vi "MarbleDispenserMk8.vi"() -> ()   [LabVIEW 2016]
uses:
  <vilib>/NXT/Block Support/NXT_InputPort.ctl
  <vilib>/NXT/Block Support/NXT_OutputPort.ctl
  <vilib>/NXT/Dual Mode Library/Sensors/Touch_Released.vi
  <vilib>/NXT/NXTIO Xnodes/NXTIONodeSubVIs/NXTStopMotors.vi
  <vilib>/NXT/NXTIO Xnodes/NXTIONodeSubVIs/NXTMotorRunDistance.vi
  <vilib>/NXT/Dual Mode Library/Waits/Wait_Num.vi
  <vilib>/NXT/Dual Mode Library/Sensors/Touch_Pressed.vi
  <vilib>/NXT/Dual Mode Library/Sensors/EV3_Color_Color.vi
  <vilib>/NXT/Dual Mode Library/Sensors/EV3_Color_Reflect.vi
  <vilib>/NXT/Subs/LVHSConnector.ctl
  <vilib>/NXT/NXTIO Xnodes/AddressXNode/NXTIOAddress.xnode
  <vilib>/NXT/NXTIO Xnodes/NXTIOXNode/NXTIO.xnode
  <vilib>/NXT/LegoClasses/BrickReference/BrickReference.lvclass
panel:
  out "Speed":dbl
  out "Color":string
  out "Distance":dbl
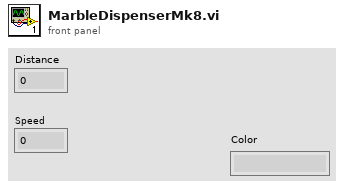
[diagram p1: front panel]
types:
  T1 = typedef "NXT_InputPort.ctl" = u32
  T2 = typedef "NXT_OutputPort.ctl" = u8
  T3 = typedef "LVHSConnector.ctl" = refnum<class "BrickReference.lvclass">
  T4 = typedef "ColorSensorColors.ctl" = enum16{"No Color", "Black", "Blue", "Green", "Yellow", "Red", "White", "Brown"}
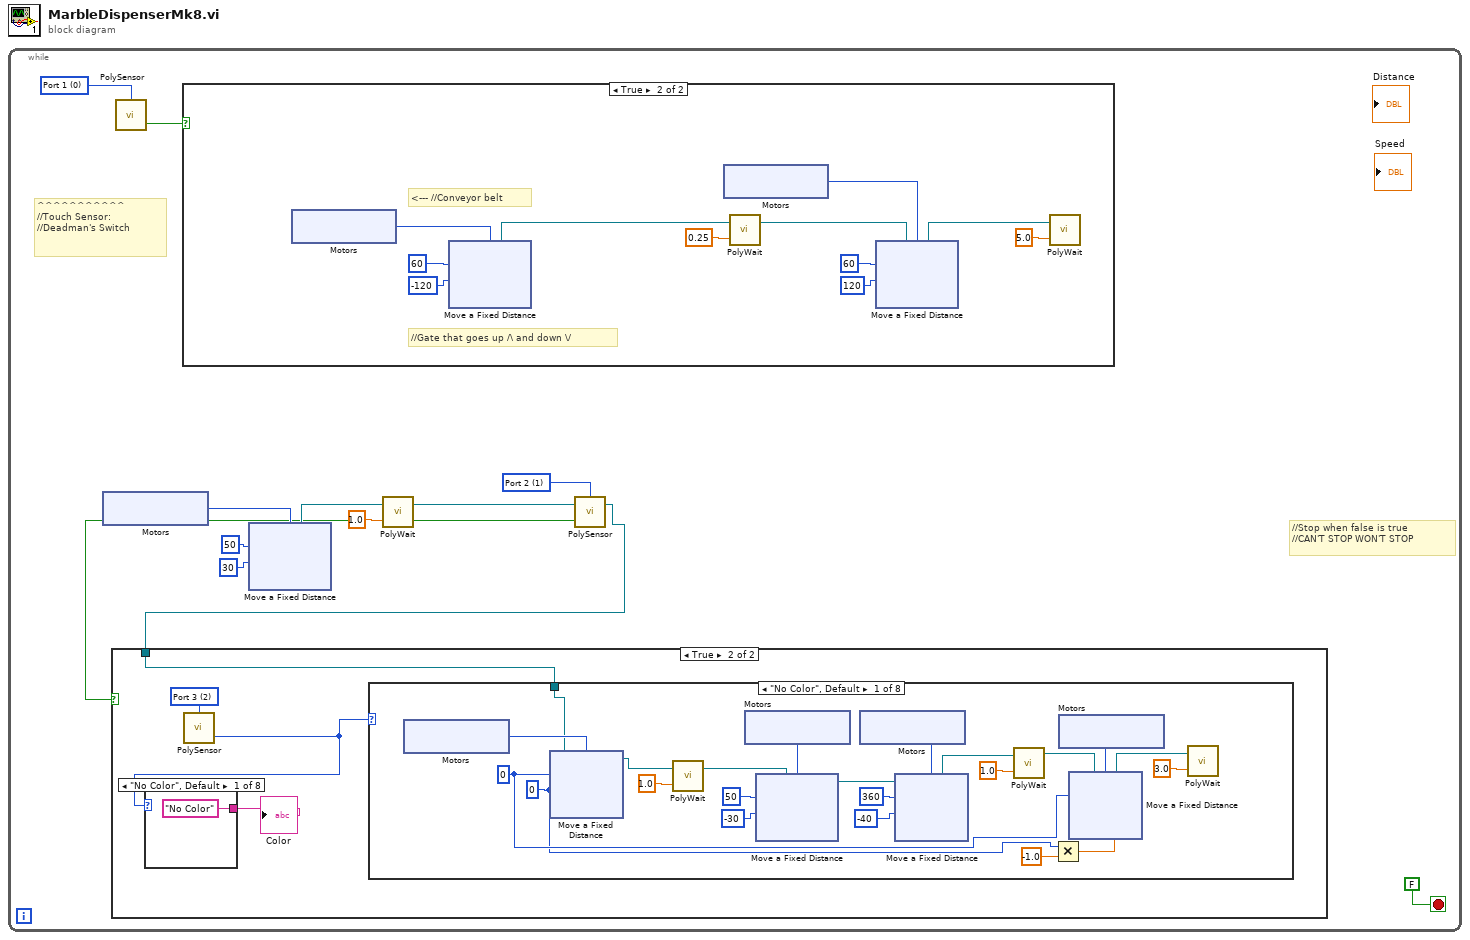
[diagram p0: block diagram]
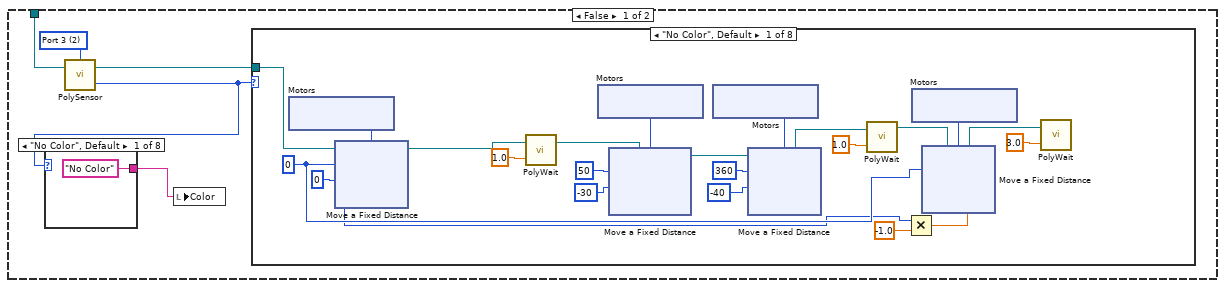
[diagram p2: hidden frame]
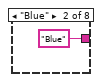
[diagram p3: hidden frame]
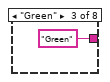
[diagram p4: hidden frame]
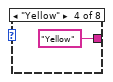
[diagram p5: hidden frame]
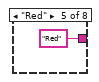
[diagram p6: hidden frame]
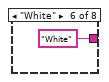
[diagram p7: hidden frame]
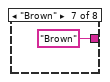
[diagram p8: hidden frame]
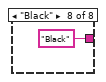
[diagram p9: hidden frame]
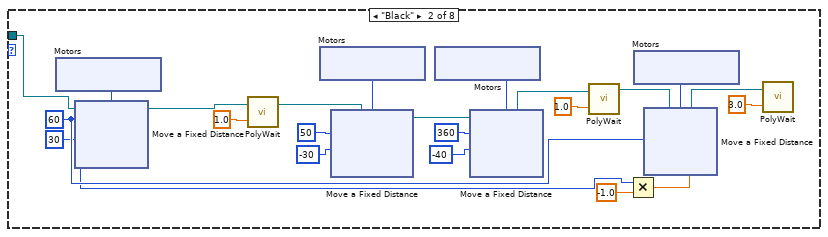
[diagram p10: hidden frame]
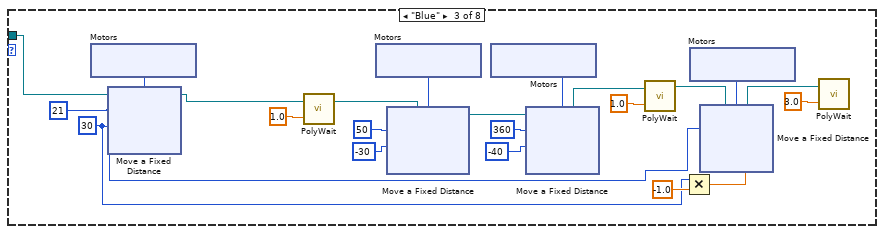
[diagram p11: hidden frame]
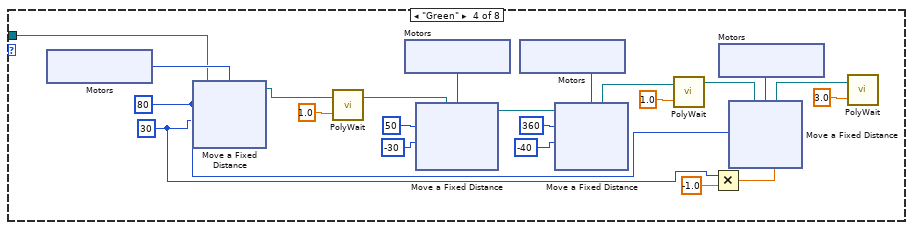
[diagram p12: hidden frame]
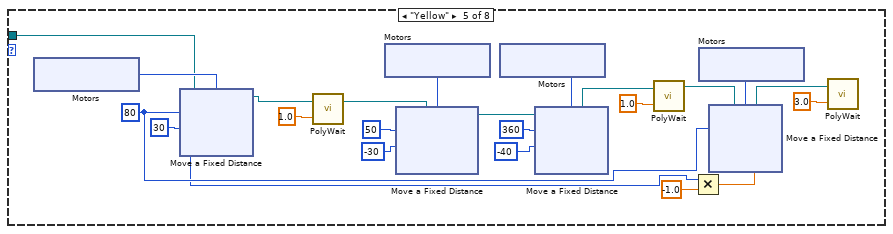
[diagram p13: hidden frame]
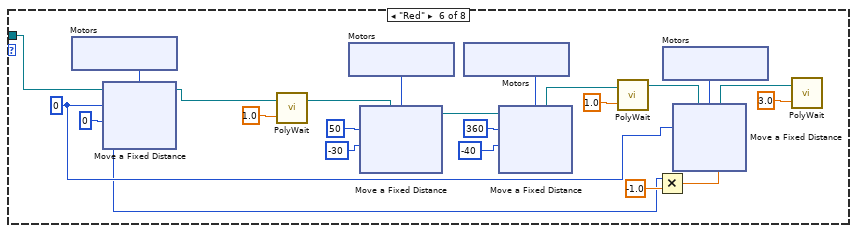
[diagram p14: hidden frame]
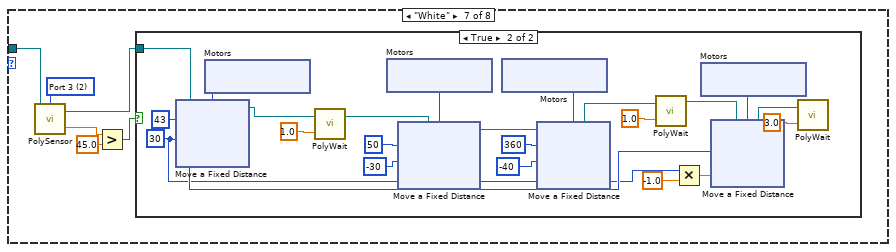
[diagram p15: hidden frame]
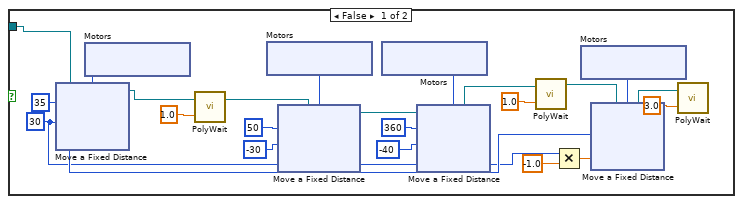
[diagram p16: hidden frame]
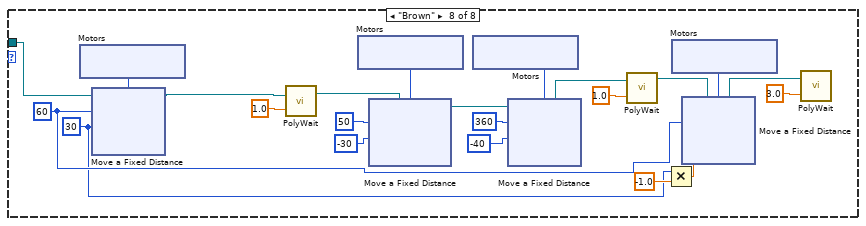
[diagram p17: hidden frame]
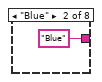
[diagram p18: hidden frame]
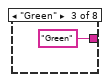
[diagram p19: hidden frame]
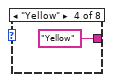
[diagram p20: hidden frame]
diagram:
  n1 = while {
    stop <- FALSE stop-if-true
    w3 = T1 1 items=["Port 1", "Port 2", "Port 3", "Port 4"] ("Port (Port 1)")
    w12 = T1 0 items=["Port 1", "Port 2", "Port 3", "Port 4"] ("Port (Port 1)")
    # "//Stop when false is true\n//CAN'T STOP WON'T STOP"
    # "^^^^^^^^^^^\n//Touch Sensor:\n//Deadman's Switch"
    n2 = xnode "Motors"() -> ("Motor"=w5:T2)
    n3 = call-poly <vilib>:"PolySensor.vi"("Port (Port 1)"=w12) -> ("Yes / No"=w10:bool)  [unwired: 2 in, 1 out]
    n4 = case shown="True" w10 {
      frame False {
        # "//This stops all the things"
        n5 = xnode "Motors"() -> ("Motor"=w1178:T2)
        n6 = xnode "Motors"() -> ("Motor"=w1177:T2)
        n7 = xnode "Stop Motors"("Motors"=w1178) -> ()  [unwired: 1 in, 1 out]
        n8 = xnode "Stop Motors"("Motors"=w1177) -> ()  [unwired: 1 in, 1 out]
      }
      frame True {
        # "//Gate that goes up /\\ and down \\/"
        # "<--- //Conveyor belt"
        n9 = xnode "Motors"() -> ("Motor"=w1197:T2)
        n10 = xnode "Move a Fixed Distance"("Speed 1"=-120, "Distance 1"=60, "Motors"=w1197) -> ("NXT/EV3"=w1200:T3)  [unwired: 1 in]
        n11 = xnode "Motors"() -> ("Motor"=w1191:T2)
        n12 = call-poly <vilib>:"PolyWait.vi"("Time (1 sec)"=0.25, "NXT/EV3"=w1200) -> ("NXT/EV3"=w1192:T3)  [unwired: 2 in]
        n13 = xnode "Move a Fixed Distance"("Speed 1"=120, "Distance 1"=60, "Motors"=w1191, "NXT/EV3"=w1192) -> ("NXT/EV3"=w1195:T3)
        n14 = call-poly <vilib>:"PolyWait.vi"("Time (1 sec)"=5.0, "NXT/EV3"=w1195) -> ()  [unwired: 2 in, 1 out]
      }
    }
    n15 = xnode "Move a Fixed Distance"("Speed 1"=30, "Distance 1"=50, "Motors"=w5) -> ("NXT/EV3"=w8:T3)  [unwired: 1 in]
    n16 = call-poly <vilib>:"PolyWait.vi"("Time (1 sec)"=1.0, "NXT/EV3"=w8) -> ("NXT/EV3"=w4:T3)  [unwired: 2 in]
    n17 = call-poly <vilib>:"PolySensor.vi"("NXT/EV3"=w4, "Port (Port 1)"=w3) -> ("Yes / No"=w2:bool, "NXT/EV3"=w1:T3)  [unwired: 1 in]
    n18 = case shown="True" w2 {
      tunnel: w1 -> [w14 w626]
      frame False {
        w17 = T1 2 items=["Port 1", "Port 2", "Port 3", "Port 4"] ("Port (Port 1)")
        n19 = call-poly <vilib>:"PolySensor.vi"("NXT/EV3"=w14, "Port (Port 1)"=w17) -> ("Detected Color"=w16:T4, "NXT/EV3"=w13:T3)  [unwired: 1 in]
        n20 = case shown="\"No Color\", Default" w16 {
          tunnel: ["No Color" "Blue" "Green" "Yellow" "Red" "White" "Brown" "Black"] -> w15
          frame "No Color", Default {
          }
          frame "Blue" {
          }
          frame "Green" {
          }
          frame "Yellow" {
          }
          frame "Red" {
          }
          frame "White" {
          }
          frame "Brown" {
          }
          frame "Black" {
          }
        }
        n21 = local write "Color"(w15) -> ()
        n22 = case shown="\"No Color\", Default" w16 {
          tunnel: w13 -> [w28 w95 w160 w227 w290 w376 w427 w560]
          frame "No Color", Default {
            w26 = i8 0 ("Speed 1")
            w27 = 0 ("Distance 1")
            n23 = xnode "Motors"() -> ("Motor"=w47:T2)
            n24 = xnode "Move a Fixed Distance"("Speed 1"=w26, "Distance 1"=w27, "Motors"=w47, "NXT/EV3"=w28) -> ("NXT/EV3"=w29:T3)
            n25 = call-poly <vilib>:"PolyWait.vi"("Time (1 sec)"=sgl 1.0, "NXT/EV3"=w29) -> ("NXT/EV3"=w42:T3)  [unwired: 2 in]
            n26 = xnode "Motors"() -> ("Motor"=w43:T2)
            n27 = xnode "Move a Fixed Distance"("Speed 1"=-30, "Distance 1"=50, "Motors"=w43, "NXT/EV3"=w42) -> ("NXT/EV3"=w32:T3)
            n28 = xnode "Motors"() -> ("Motor"=w39:T2)
            n29 = xnode "Move a Fixed Distance"("Speed 1"=i8 -40, "Distance 1"=360, "Motors"=w39, "NXT/EV3"=w32) -> ("NXT/EV3"=w40:T3)
            n30 = call-poly <vilib>:"PolyWait.vi"("Time (1 sec)"=1.0, "NXT/EV3"=w40) -> ("NXT/EV3"=w35:T3)  [unwired: 2 in]
            n31 = Multiply(x=w26, y=-1.0) -> (x*y=w30:dbl)
            n32 = xnode "Motors"() -> ("Motor"=w34:T2)
            n33 = xnode "Move a Fixed Distance"("Speed 1"=w30, "Distance 1"=w27, "Motors"=w34, "NXT/EV3"=w35) -> ("NXT/EV3"=w33:T3)
            n34 = call-poly <vilib>:"PolyWait.vi"("Time (1 sec)"=3.0, "NXT/EV3"=w33) -> ()  [unwired: 2 in, 1 out]
          }
          frame "Black" {
            w92 = i8 30 ("Speed 1")
            w93 = 60 ("Distance 1")
            n35 = xnode "Motors"() -> ("Motor"=w113:T2)
            n36 = xnode "Move a Fixed Distance"("Speed 1"=w92, "Distance 1"=w93, "Motors"=w113, "NXT/EV3"=w95) -> ("NXT/EV3"=w94:T3)
            n37 = call-poly <vilib>:"PolyWait.vi"("Time (1 sec)"=sgl 1.0, "NXT/EV3"=w94) -> ("NXT/EV3"=w108:T3)  [unwired: 2 in]
            n38 = xnode "Motors"() -> ("Motor"=w109:T2)
            n39 = xnode "Move a Fixed Distance"("Speed 1"=-30, "Distance 1"=50, "Motors"=w109, "NXT/EV3"=w108) -> ("NXT/EV3"=w98:T3)
            n40 = xnode "Motors"() -> ("Motor"=w105:T2)
            n41 = xnode "Move a Fixed Distance"("Speed 1"=i8 -40, "Distance 1"=360, "Motors"=w105, "NXT/EV3"=w98) -> ("NXT/EV3"=w106:T3)
            n42 = call-poly <vilib>:"PolyWait.vi"("Time (1 sec)"=1.0, "NXT/EV3"=w106) -> ("NXT/EV3"=w101:T3)  [unwired: 2 in]
            n43 = Multiply(x=w92, y=-1.0) -> (x*y=w96:dbl)
            n44 = xnode "Motors"() -> ("Motor"=w100:T2)
            n45 = xnode "Move a Fixed Distance"("Speed 1"=w96, "Distance 1"=w93, "Motors"=w100, "NXT/EV3"=w101) -> ("NXT/EV3"=w99:T3)
            n46 = call-poly <vilib>:"PolyWait.vi"("Time (1 sec)"=3.0, "NXT/EV3"=w99) -> ()  [unwired: 2 in, 1 out]
          }
          frame "Blue" {
            w158 = i8 30 ("Speed 1")
            w159 = 21 ("Distance 1")
            n47 = xnode "Motors"() -> ("Motor"=w179:T2)
            n48 = xnode "Move a Fixed Distance"("Speed 1"=w158, "Distance 1"=w159, "Motors"=w179, "NXT/EV3"=w160) -> ("NXT/EV3"=w161:T3)
            n49 = call-poly <vilib>:"PolyWait.vi"("Time (1 sec)"=sgl 1.0, "NXT/EV3"=w161) -> ("NXT/EV3"=w174:T3)  [unwired: 2 in]
            n50 = xnode "Motors"() -> ("Motor"=w175:T2)
            n51 = xnode "Move a Fixed Distance"("Speed 1"=-30, "Distance 1"=50, "Motors"=w175, "NXT/EV3"=w174) -> ("NXT/EV3"=w164:T3)
            n52 = xnode "Motors"() -> ("Motor"=w171:T2)
            n53 = xnode "Move a Fixed Distance"("Speed 1"=i8 -40, "Distance 1"=360, "Motors"=w171, "NXT/EV3"=w164) -> ("NXT/EV3"=w172:T3)
            n54 = call-poly <vilib>:"PolyWait.vi"("Time (1 sec)"=1.0, "NXT/EV3"=w172) -> ("NXT/EV3"=w167:T3)  [unwired: 2 in]
            n55 = Multiply(x=w158, y=-1.0) -> (x*y=w162:dbl)
            n56 = xnode "Motors"() -> ("Motor"=w166:T2)
            n57 = xnode "Move a Fixed Distance"("Speed 1"=w162, "Distance 1"=w159, "Motors"=w166, "NXT/EV3"=w167) -> ("NXT/EV3"=w165:T3)
            n58 = call-poly <vilib>:"PolyWait.vi"("Time (1 sec)"=3.0, "NXT/EV3"=w165) -> ()  [unwired: 2 in, 1 out]
          }
          frame "Green" {
            w224 = i8 30 ("Speed 1")
            w225 = 80 ("Distance 1")
            n59 = xnode "Motors"() -> ("Motor"=w245:T2)
            n60 = xnode "Move a Fixed Distance"("Speed 1"=w224, "Distance 1"=w225, "Motors"=w245, "NXT/EV3"=w227) -> ("NXT/EV3"=w226:T3)
            n61 = call-poly <vilib>:"PolyWait.vi"("Time (1 sec)"=sgl 1.0, "NXT/EV3"=w226) -> ("NXT/EV3"=w240:T3)  [unwired: 2 in]
            n62 = xnode "Motors"() -> ("Motor"=w241:T2)
            n63 = xnode "Move a Fixed Distance"("Speed 1"=-30, "Distance 1"=50, "Motors"=w241, "NXT/EV3"=w240) -> ("NXT/EV3"=w230:T3)
            n64 = xnode "Motors"() -> ("Motor"=w237:T2)
            n65 = xnode "Move a Fixed Distance"("Speed 1"=i8 -40, "Distance 1"=360, "Motors"=w237, "NXT/EV3"=w230) -> ("NXT/EV3"=w238:T3)
            n66 = call-poly <vilib>:"PolyWait.vi"("Time (1 sec)"=1.0, "NXT/EV3"=w238) -> ("NXT/EV3"=w233:T3)  [unwired: 2 in]
            n67 = Multiply(x=w224, y=-1.0) -> (x*y=w228:dbl)
            n68 = xnode "Motors"() -> ("Motor"=w232:T2)
            n69 = xnode "Move a Fixed Distance"("Speed 1"=w228, "Distance 1"=w225, "Motors"=w232, "NXT/EV3"=w233) -> ("NXT/EV3"=w231:T3)
            n70 = call-poly <vilib>:"PolyWait.vi"("Time (1 sec)"=3.0, "NXT/EV3"=w231) -> ()  [unwired: 2 in, 1 out]
          }
          frame "Yellow" {
            w291 = i8 30 ("Speed 1")
            w292 = 80 ("Distance 1")
            n71 = xnode "Motors"() -> ("Motor"=w311:T2)
            n72 = xnode "Move a Fixed Distance"("Speed 1"=w291, "Distance 1"=w292, "Motors"=w311, "NXT/EV3"=w290) -> ("NXT/EV3"=w293:T3)
            n73 = call-poly <vilib>:"PolyWait.vi"("Time (1 sec)"=sgl 1.0, "NXT/EV3"=w293) -> ("NXT/EV3"=w306:T3)  [unwired: 2 in]
            n74 = xnode "Motors"() -> ("Motor"=w307:T2)
            n75 = xnode "Move a Fixed Distance"("Speed 1"=-30, "Distance 1"=50, "Motors"=w307, "NXT/EV3"=w306) -> ("NXT/EV3"=w296:T3)
            n76 = xnode "Motors"() -> ("Motor"=w303:T2)
            n77 = xnode "Move a Fixed Distance"("Speed 1"=i8 -40, "Distance 1"=360, "Motors"=w303, "NXT/EV3"=w296) -> ("NXT/EV3"=w304:T3)
            n78 = call-poly <vilib>:"PolyWait.vi"("Time (1 sec)"=1.0, "NXT/EV3"=w304) -> ("NXT/EV3"=w299:T3)  [unwired: 2 in]
            n79 = Multiply(x=w291, y=-1.0) -> (x*y=w294:dbl)
            n80 = xnode "Motors"() -> ("Motor"=w298:T2)
            n81 = xnode "Move a Fixed Distance"("Speed 1"=w294, "Distance 1"=w292, "Motors"=w298, "NXT/EV3"=w299) -> ("NXT/EV3"=w297:T3)
            n82 = call-poly <vilib>:"PolyWait.vi"("Time (1 sec)"=3.0, "NXT/EV3"=w297) -> ()  [unwired: 2 in, 1 out]
          }
          frame "Red" {
            w356 = i8 0 ("Speed 1")
            w357 = 0 ("Distance 1")
            n83 = xnode "Motors"() -> ("Motor"=w377:T2)
            n84 = xnode "Move a Fixed Distance"("Speed 1"=w356, "Distance 1"=w357, "Motors"=w377, "NXT/EV3"=w376) -> ("NXT/EV3"=w358:T3)
            n85 = call-poly <vilib>:"PolyWait.vi"("Time (1 sec)"=sgl 1.0, "NXT/EV3"=w358) -> ("NXT/EV3"=w371:T3)  [unwired: 2 in]
            n86 = xnode "Motors"() -> ("Motor"=w372:T2)
            n87 = xnode "Move a Fixed Distance"("Speed 1"=-30, "Distance 1"=50, "Motors"=w372, "NXT/EV3"=w371) -> ("NXT/EV3"=w361:T3)
            n88 = xnode "Motors"() -> ("Motor"=w368:T2)
            n89 = xnode "Move a Fixed Distance"("Speed 1"=i8 -40, "Distance 1"=360, "Motors"=w368, "NXT/EV3"=w361) -> ("NXT/EV3"=w369:T3)
            n90 = call-poly <vilib>:"PolyWait.vi"("Time (1 sec)"=1.0, "NXT/EV3"=w369) -> ("NXT/EV3"=w364:T3)  [unwired: 2 in]
            n91 = Multiply(x=w356, y=-1.0) -> (x*y=w359:dbl)
            n92 = xnode "Motors"() -> ("Motor"=w363:T2)
            n93 = xnode "Move a Fixed Distance"("Speed 1"=w359, "Distance 1"=w357, "Motors"=w363, "NXT/EV3"=w364) -> ("NXT/EV3"=w362:T3)
            n94 = call-poly <vilib>:"PolyWait.vi"("Time (1 sec)"=3.0, "NXT/EV3"=w362) -> ()  [unwired: 2 in, 1 out]
          }
          frame "White" {
            w425 = T1 2 items=["Port 1", "Port 2", "Port 3", "Port 4"] ("Port (Port 1)")
            n95 = call-poly <vilib>:"PolySensor.vi"("NXT/EV3"=w427, "Port (Port 1)"=w425) -> ("Scaled Value"=w424:sgl, "NXT/EV3"=w426:T3)  [unwired: 1 in]
            n96 = Greater?(x=w424, y=sgl 45.0) -> (0:w422:bool)
            n97 = case shown="True" w422 {
              tunnel: w426 -> [w428 w514]
              frame False {
                w429 = i8 30 ("Speed 1")
                w430 = 35 ("Distance 1")
                n98 = xnode "Motors"() -> ("Motor"=w449:T2)
                n99 = xnode "Move a Fixed Distance"("Speed 1"=w429, "Distance 1"=w430, "Motors"=w449, "NXT/EV3"=w428) -> ("NXT/EV3"=w431:T3)
                n100 = call-poly <vilib>:"PolyWait.vi"("Time (1 sec)"=sgl 1.0, "NXT/EV3"=w431) -> ("NXT/EV3"=w444:T3)  [unwired: 2 in]
                n101 = xnode "Motors"() -> ("Motor"=w445:T2)
                n102 = xnode "Move a Fixed Distance"("Speed 1"=-30, "Distance 1"=50, "Motors"=w445, "NXT/EV3"=w444) -> ("NXT/EV3"=w434:T3)
                n103 = xnode "Motors"() -> ("Motor"=w441:T2)
                n104 = xnode "Move a Fixed Distance"("Speed 1"=i8 -40, "Distance 1"=360, "Motors"=w441, "NXT/EV3"=w434) -> ("NXT/EV3"=w442:T3)
                n105 = call-poly <vilib>:"PolyWait.vi"("Time (1 sec)"=1.0, "NXT/EV3"=w442) -> ("NXT/EV3"=w437:T3)  [unwired: 2 in]
                n106 = Multiply(x=w429, y=-1.0) -> (x*y=w432:dbl)
                n107 = xnode "Motors"() -> ("Motor"=w436:T2)
                n108 = xnode "Move a Fixed Distance"("Speed 1"=w432, "Distance 1"=w430, "Motors"=w436, "NXT/EV3"=w437) -> ("NXT/EV3"=w435:T3)
                n109 = call-poly <vilib>:"PolyWait.vi"("Time (1 sec)"=3.0, "NXT/EV3"=w435) -> ()  [unwired: 2 in, 1 out]
              }
              frame True {
                w494 = i8 30 ("Speed 1")
                w495 = 43 ("Distance 1")
                n110 = xnode "Motors"() -> ("Motor"=w515:T2)
                n111 = xnode "Move a Fixed Distance"("Speed 1"=w494, "Distance 1"=w495, "Motors"=w515, "NXT/EV3"=w514) -> ("NXT/EV3"=w496:T3)
                n112 = call-poly <vilib>:"PolyWait.vi"("Time (1 sec)"=sgl 1.0, "NXT/EV3"=w496) -> ("NXT/EV3"=w509:T3)  [unwired: 2 in]
                n113 = xnode "Motors"() -> ("Motor"=w510:T2)
                n114 = xnode "Move a Fixed Distance"("Speed 1"=-30, "Distance 1"=50, "Motors"=w510, "NXT/EV3"=w509) -> ("NXT/EV3"=w499:T3)
                n115 = xnode "Motors"() -> ("Motor"=w506:T2)
                n116 = xnode "Move a Fixed Distance"("Speed 1"=i8 -40, "Distance 1"=360, "Motors"=w506, "NXT/EV3"=w499) -> ("NXT/EV3"=w507:T3)
                n117 = call-poly <vilib>:"PolyWait.vi"("Time (1 sec)"=1.0, "NXT/EV3"=w507) -> ("NXT/EV3"=w502:T3)  [unwired: 2 in]
                n118 = Multiply(x=w494, y=-1.0) -> (x*y=w497:dbl)
                n119 = xnode "Motors"() -> ("Motor"=w501:T2)
                n120 = xnode "Move a Fixed Distance"("Speed 1"=w497, "Distance 1"=w495, "Motors"=w501, "NXT/EV3"=w502) -> ("NXT/EV3"=w500:T3)
                n121 = call-poly <vilib>:"PolyWait.vi"("Time (1 sec)"=3.0, "NXT/EV3"=w500) -> ()  [unwired: 2 in, 1 out]
              }
            }
          }
          frame "Brown" {
            w561 = i8 30 ("Speed 1")
            w562 = 60 ("Distance 1")
            n122 = xnode "Motors"() -> ("Motor"=w581:T2)
            n123 = xnode "Move a Fixed Distance"("Speed 1"=w561, "Distance 1"=w562, "Motors"=w581, "NXT/EV3"=w560) -> ("NXT/EV3"=w563:T3)
            n124 = call-poly <vilib>:"PolyWait.vi"("Time (1 sec)"=sgl 1.0, "NXT/EV3"=w563) -> ("NXT/EV3"=w576:T3)  [unwired: 2 in]
            n125 = xnode "Motors"() -> ("Motor"=w577:T2)
            n126 = xnode "Move a Fixed Distance"("Speed 1"=-30, "Distance 1"=50, "Motors"=w577, "NXT/EV3"=w576) -> ("NXT/EV3"=w566:T3)
            n127 = xnode "Motors"() -> ("Motor"=w573:T2)
            n128 = xnode "Move a Fixed Distance"("Speed 1"=i8 -40, "Distance 1"=360, "Motors"=w573, "NXT/EV3"=w566) -> ("NXT/EV3"=w574:T3)
            n129 = call-poly <vilib>:"PolyWait.vi"("Time (1 sec)"=1.0, "NXT/EV3"=w574) -> ("NXT/EV3"=w569:T3)  [unwired: 2 in]
            n130 = Multiply(x=w561, y=-1.0) -> (x*y=w564:dbl)
            n131 = xnode "Motors"() -> ("Motor"=w568:T2)
            n132 = xnode "Move a Fixed Distance"("Speed 1"=w564, "Distance 1"=w562, "Motors"=w568, "NXT/EV3"=w569) -> ("NXT/EV3"=w567:T3)
            n133 = call-poly <vilib>:"PolyWait.vi"("Time (1 sec)"=3.0, "NXT/EV3"=w567) -> ()  [unwired: 2 in, 1 out]
          }
        }
      }
      frame True {
        w629 = T1 2 items=["Port 1", "Port 2", "Port 3", "Port 4"] ("Port (Port 1)")
        n134 = call-poly <vilib>:"PolySensor.vi"("Port (Port 1)"=w629) -> ("Detected Color"=w627:T4)  [unwired: 2 in, 1 out]
        n135 = case shown="\"No Color\", Default" w627 {
          tunnel: ["No Color" "Blue" "Green" "Yellow" "Red" "White" "Brown" "Black"] -> w628
          frame "No Color", Default {
          }
          frame "Blue" {
          }
          frame "Green" {
          }
          frame "Yellow" {
          }
          frame "Red" {
          }
          frame "White" {
          }
          frame "Brown" {
          }
          frame "Black" {
          }
        }
        "Color" <- w628
        n136 = case shown="\"No Color\", Default" w627 {
          tunnel: w626 -> [w640 w706 w790 w856 w904 w988 w1036 w1102]
          frame "No Color", Default {
            w638 = i8 0 ("Speed 1")
            w639 = 0 ("Distance 1")
            n137 = xnode "Motors"() -> ("Motor"=w659:T2)
            n138 = xnode "Move a Fixed Distance"("Speed 1"=w638, "Distance 1"=w639, "Motors"=w659, "NXT/EV3"=w640) -> ("NXT/EV3"=w641:T3)
            n139 = call-poly <vilib>:"PolyWait.vi"("Time (1 sec)"=sgl 1.0, "NXT/EV3"=w641) -> ("NXT/EV3"=w654:T3)  [unwired: 2 in]
            n140 = xnode "Motors"() -> ("Motor"=w655:T2)
            n141 = xnode "Move a Fixed Distance"("Speed 1"=-30, "Distance 1"=50, "Motors"=w655, "NXT/EV3"=w654) -> ("NXT/EV3"=w644:T3)
            n142 = xnode "Motors"() -> ("Motor"=w651:T2)
            n143 = xnode "Move a Fixed Distance"("Speed 1"=i8 -40, "Distance 1"=360, "Motors"=w651, "NXT/EV3"=w644) -> ("NXT/EV3"=w652:T3)
            n144 = call-poly <vilib>:"PolyWait.vi"("Time (1 sec)"=1.0, "NXT/EV3"=w652) -> ("NXT/EV3"=w647:T3)  [unwired: 2 in]
            n145 = Multiply(x=w638, y=-1.0) -> (x*y=w642:dbl)
            n146 = xnode "Motors"() -> ("Motor"=w646:T2)
            n147 = xnode "Move a Fixed Distance"("Speed 1"=w642, "Distance 1"=w639, "Motors"=w646, "NXT/EV3"=w647) -> ("NXT/EV3"=w645:T3)
            n148 = call-poly <vilib>:"PolyWait.vi"("Time (1 sec)"=3.0, "NXT/EV3"=w645) -> ()  [unwired: 2 in, 1 out]
          }
          frame "Black" {
            w704 = i8 30 ("Speed 1")
            w705 = 10 ("Distance 1")
            n149 = xnode "Motors"() -> ("Motor"=w725:T2)
            n150 = xnode "Move a Fixed Distance"("Speed 1"=w704, "Distance 1"=w705, "Motors"=w725, "NXT/EV3"=w706) -> ("NXT/EV3"=w707:T3)
            n151 = call-poly <vilib>:"PolyWait.vi"("Time (1 sec)"=sgl 1.0, "NXT/EV3"=w707) -> ("NXT/EV3"=w720:T3)  [unwired: 2 in]
            n152 = xnode "Motors"() -> ("Motor"=w721:T2)
            n153 = xnode "Move a Fixed Distance"("Speed 1"=-30, "Distance 1"=50, "Motors"=w721, "NXT/EV3"=w720) -> ("NXT/EV3"=w710:T3)
            n154 = xnode "Motors"() -> ("Motor"=w717:T2)
            n155 = xnode "Move a Fixed Distance"("Speed 1"=i8 -40, "Distance 1"=360, "Motors"=w717, "NXT/EV3"=w710) -> ("NXT/EV3"=w718:T3)
            n156 = call-poly <vilib>:"PolyWait.vi"("Time (1 sec)"=1.0, "NXT/EV3"=w718) -> ("NXT/EV3"=w713:T3)  [unwired: 2 in]
            n157 = Multiply(x=w704, y=-1.0) -> (x*y=w708:dbl)
            n158 = xnode "Motors"() -> ("Motor"=w712:T2)
            n159 = xnode "Move a Fixed Distance"("Speed 1"=w708, "Distance 1"=w705, "Motors"=w712, "NXT/EV3"=w713) -> ("NXT/EV3"=w711:T3)
            n160 = call-poly <vilib>:"PolyWait.vi"("Time (1 sec)"=3.0, "NXT/EV3"=w711) -> ()  [unwired: 2 in, 1 out]
          }
          frame "Blue" {
            w770 = i8 30 ("Speed 1")
            w771 = 32 ("Distance 1")
            n161 = xnode "Motors"() -> ("Motor"=w791:T2)
            n162 = xnode "Move a Fixed Distance"("Speed 1"=w770, "Distance 1"=w771, "Motors"=w791, "NXT/EV3"=w790) -> ("NXT/EV3"=w772:T3)
            n163 = call-poly <vilib>:"PolyWait.vi"("Time (1 sec)"=sgl 1.0, "NXT/EV3"=w772) -> ("NXT/EV3"=w785:T3)  [unwired: 2 in]
            n164 = xnode "Motors"() -> ("Motor"=w786:T2)
            n165 = xnode "Move a Fixed Distance"("Speed 1"=-30, "Distance 1"=50, "Motors"=w786, "NXT/EV3"=w785) -> ("NXT/EV3"=w775:T3)
            n166 = xnode "Motors"() -> ("Motor"=w782:T2)
            n167 = xnode "Move a Fixed Distance"("Speed 1"=i8 -40, "Distance 1"=360, "Motors"=w782, "NXT/EV3"=w775) -> ("NXT/EV3"=w783:T3)
            n168 = call-poly <vilib>:"PolyWait.vi"("Time (1 sec)"=1.0, "NXT/EV3"=w783) -> ("NXT/EV3"=w778:T3)  [unwired: 2 in]
            n169 = Multiply(x=w770, y=-1.0) -> (x*y=w773:dbl)
            n170 = xnode "Motors"() -> ("Motor"=w777:T2)
            n171 = xnode "Move a Fixed Distance"("Speed 1"=w773, "Distance 1"=w771, "Motors"=w777, "NXT/EV3"=w778) -> ("NXT/EV3"=w776:T3)
            n172 = call-poly <vilib>:"PolyWait.vi"("Time (1 sec)"=3.0, "NXT/EV3"=w776) -> ()  [unwired: 2 in, 1 out]
          }
          frame "Green" {
            w836 = i8 30 ("Speed 1")
            w837 = 80 ("Distance 1")
            n173 = xnode "Motors"() -> ("Motor"=w857:T2)
            n174 = xnode "Move a Fixed Distance"("Speed 1"=w836, "Distance 1"=w837, "Motors"=w857, "NXT/EV3"=w856) -> ("NXT/EV3"=w838:T3)
            n175 = call-poly <vilib>:"PolyWait.vi"("Time (1 sec)"=sgl 1.0, "NXT/EV3"=w838) -> ("NXT/EV3"=w851:T3)  [unwired: 2 in]
            n176 = xnode "Motors"() -> ("Motor"=w852:T2)
            n177 = xnode "Move a Fixed Distance"("Speed 1"=-30, "Distance 1"=50, "Motors"=w852, "NXT/EV3"=w851) -> ("NXT/EV3"=w841:T3)
            n178 = xnode "Motors"() -> ("Motor"=w848:T2)
            n179 = xnode "Move a Fixed Distance"("Speed 1"=i8 -40, "Distance 1"=360, "Motors"=w848, "NXT/EV3"=w841) -> ("NXT/EV3"=w849:T3)
            n180 = call-poly <vilib>:"PolyWait.vi"("Time (1 sec)"=1.0, "NXT/EV3"=w849) -> ("NXT/EV3"=w844:T3)  [unwired: 2 in]
            n181 = Multiply(x=w836, y=-1.0) -> (x*y=w839:dbl)
            n182 = xnode "Motors"() -> ("Motor"=w843:T2)
            n183 = xnode "Move a Fixed Distance"("Speed 1"=w839, "Distance 1"=w837, "Motors"=w843, "NXT/EV3"=w844) -> ("NXT/EV3"=w842:T3)
            n184 = call-poly <vilib>:"PolyWait.vi"("Time (1 sec)"=3.0, "NXT/EV3"=w842) -> ()  [unwired: 2 in, 1 out]
          }
          frame "Yellow" {
            w902 = i8 30 ("Speed 1")
            w903 = 80 ("Distance 1")
            n185 = xnode "Motors"() -> ("Motor"=w923:T2)
            n186 = xnode "Move a Fixed Distance"("Speed 1"=w902, "Distance 1"=w903, "Motors"=w923, "NXT/EV3"=w904) -> ("NXT/EV3"=w905:T3)
            n187 = call-poly <vilib>:"PolyWait.vi"("Time (1 sec)"=sgl 1.0, "NXT/EV3"=w905) -> ("NXT/EV3"=w918:T3)  [unwired: 2 in]
            n188 = xnode "Motors"() -> ("Motor"=w919:T2)
            n189 = xnode "Move a Fixed Distance"("Speed 1"=-30, "Distance 1"=50, "Motors"=w919, "NXT/EV3"=w918) -> ("NXT/EV3"=w908:T3)
            n190 = xnode "Motors"() -> ("Motor"=w915:T2)
            n191 = xnode "Move a Fixed Distance"("Speed 1"=i8 -40, "Distance 1"=360, "Motors"=w915, "NXT/EV3"=w908) -> ("NXT/EV3"=w916:T3)
            n192 = call-poly <vilib>:"PolyWait.vi"("Time (1 sec)"=1.0, "NXT/EV3"=w916) -> ("NXT/EV3"=w911:T3)  [unwired: 2 in]
            n193 = Multiply(x=w902, y=-1.0) -> (x*y=w906:dbl)
            n194 = xnode "Motors"() -> ("Motor"=w910:T2)
            n195 = xnode "Move a Fixed Distance"("Speed 1"=w906, "Distance 1"=w903, "Motors"=w910, "NXT/EV3"=w911) -> ("NXT/EV3"=w909:T3)
            n196 = call-poly <vilib>:"PolyWait.vi"("Time (1 sec)"=3.0, "NXT/EV3"=w909) -> ()  [unwired: 2 in, 1 out]
          }
          frame "Red" {
            w968 = i8 30 ("Speed 1")
            w969 = 10 ("Distance 1")
            n197 = xnode "Motors"() -> ("Motor"=w989:T2)
            n198 = xnode "Move a Fixed Distance"("Speed 1"=w968, "Distance 1"=w969, "Motors"=w989, "NXT/EV3"=w988) -> ("NXT/EV3"=w970:T3)
            n199 = call-poly <vilib>:"PolyWait.vi"("Time (1 sec)"=sgl 1.0, "NXT/EV3"=w970) -> ("NXT/EV3"=w983:T3)  [unwired: 2 in]
            n200 = xnode "Motors"() -> ("Motor"=w984:T2)
            n201 = xnode "Move a Fixed Distance"("Speed 1"=-30, "Distance 1"=50, "Motors"=w984, "NXT/EV3"=w983) -> ("NXT/EV3"=w973:T3)
            n202 = xnode "Motors"() -> ("Motor"=w980:T2)
            n203 = xnode "Move a Fixed Distance"("Speed 1"=i8 -40, "Distance 1"=360, "Motors"=w980, "NXT/EV3"=w973) -> ("NXT/EV3"=w981:T3)
            n204 = call-poly <vilib>:"PolyWait.vi"("Time (1 sec)"=1.0, "NXT/EV3"=w981) -> ("NXT/EV3"=w976:T3)  [unwired: 2 in]
            n205 = Multiply(x=w968, y=-1.0) -> (x*y=w971:dbl)
            n206 = xnode "Motors"() -> ("Motor"=w975:T2)
            n207 = xnode "Move a Fixed Distance"("Speed 1"=w971, "Distance 1"=w969, "Motors"=w975, "NXT/EV3"=w976) -> ("NXT/EV3"=w974:T3)
            n208 = call-poly <vilib>:"PolyWait.vi"("Time (1 sec)"=3.0, "NXT/EV3"=w974) -> ()  [unwired: 2 in, 1 out]
          }
          frame "White" {
            w1034 = i8 30 ("Speed 1")
            w1035 = 73 ("Distance 1")
            n209 = xnode "Motors"() -> ("Motor"=w1055:T2)
            n210 = xnode "Move a Fixed Distance"("Speed 1"=w1034, "Distance 1"=w1035, "Motors"=w1055, "NXT/EV3"=w1036) -> ("NXT/EV3"=w1037:T3)
            n211 = call-poly <vilib>:"PolyWait.vi"("Time (1 sec)"=sgl 1.0, "NXT/EV3"=w1037) -> ("NXT/EV3"=w1050:T3)  [unwired: 2 in]
            n212 = xnode "Motors"() -> ("Motor"=w1051:T2)
            n213 = xnode "Move a Fixed Distance"("Speed 1"=-30, "Distance 1"=50, "Motors"=w1051, "NXT/EV3"=w1050) -> ("NXT/EV3"=w1040:T3)
            n214 = xnode "Motors"() -> ("Motor"=w1047:T2)
            n215 = xnode "Move a Fixed Distance"("Speed 1"=i8 -40, "Distance 1"=360, "Motors"=w1047, "NXT/EV3"=w1040) -> ("NXT/EV3"=w1048:T3)
            n216 = call-poly <vilib>:"PolyWait.vi"("Time (1 sec)"=1.0, "NXT/EV3"=w1048) -> ("NXT/EV3"=w1043:T3)  [unwired: 2 in]
            n217 = Multiply(x=w1034, y=-1.0) -> (x*y=w1038:dbl)
            n218 = xnode "Motors"() -> ("Motor"=w1042:T2)
            n219 = xnode "Move a Fixed Distance"("Speed 1"=w1038, "Distance 1"=w1035, "Motors"=w1042, "NXT/EV3"=w1043) -> ("NXT/EV3"=w1041:T3)
            n220 = call-poly <vilib>:"PolyWait.vi"("Time (1 sec)"=3.0, "NXT/EV3"=w1041) -> ()  [unwired: 2 in, 1 out]
          }
          frame "Brown" {
            w1100 = i8 30 ("Speed 1")
            w1101 = 10 ("Distance 1")
            n221 = xnode "Motors"() -> ("Motor"=w1121:T2)
            n222 = xnode "Move a Fixed Distance"("Speed 1"=w1100, "Distance 1"=w1101, "Motors"=w1121, "NXT/EV3"=w1102) -> ("NXT/EV3"=w1103:T3)
            n223 = call-poly <vilib>:"PolyWait.vi"("Time (1 sec)"=sgl 1.0, "NXT/EV3"=w1103) -> ("NXT/EV3"=w1116:T3)  [unwired: 2 in]
            n224 = xnode "Motors"() -> ("Motor"=w1117:T2)
            n225 = xnode "Move a Fixed Distance"("Speed 1"=-30, "Distance 1"=50, "Motors"=w1117, "NXT/EV3"=w1116) -> ("NXT/EV3"=w1106:T3)
            n226 = xnode "Motors"() -> ("Motor"=w1113:T2)
            n227 = xnode "Move a Fixed Distance"("Speed 1"=i8 -40, "Distance 1"=360, "Motors"=w1113, "NXT/EV3"=w1106) -> ("NXT/EV3"=w1114:T3)
            n228 = call-poly <vilib>:"PolyWait.vi"("Time (1 sec)"=1.0, "NXT/EV3"=w1114) -> ("NXT/EV3"=w1109:T3)  [unwired: 2 in]
            n229 = Multiply(x=w1100, y=-1.0) -> (x*y=w1104:dbl)
            n230 = xnode "Motors"() -> ("Motor"=w1108:T2)
            n231 = xnode "Move a Fixed Distance"("Speed 1"=w1104, "Distance 1"=w1101, "Motors"=w1108, "NXT/EV3"=w1109) -> ("NXT/EV3"=w1107:T3)
            n232 = call-poly <vilib>:"PolyWait.vi"("Time (1 sec)"=3.0, "NXT/EV3"=w1107) -> ()  [unwired: 2 in, 1 out]
          }
        }
      }
    }
  }
